vi "AIDI-Initialize DI.vi"(0 "DI":T2, 7 "Sync Task":refnum<k21>, 11 "error in (no error)":errorcluster) -> (4 "DI Tasks":T1, 15 "error out":errorcluster)   [LabVIEW 2020]
uses:
  Typedefs/DI-Output Spec.ctl
  Typedefs/AIDI-DI Tasks.ctl
  <resource>/objmgr/daqmx.rc
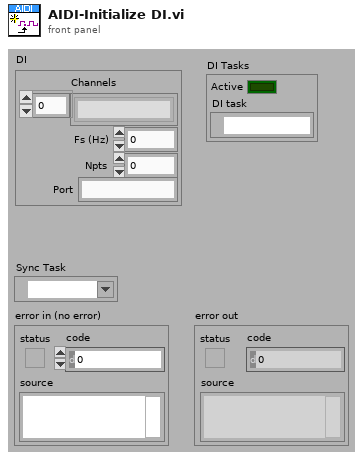
[diagram p1: front panel]
types:
  T1 = typedef "AIDI-DI Tasks.ctl" = cluster{"Active":bool, "DI task":refnum<k21>}
  T2 = typedef "DI-Output Spec.ctl" = cluster{"Channels":string[], "Fs (Hz)":dbl, "Npts":i32, "Port":string}
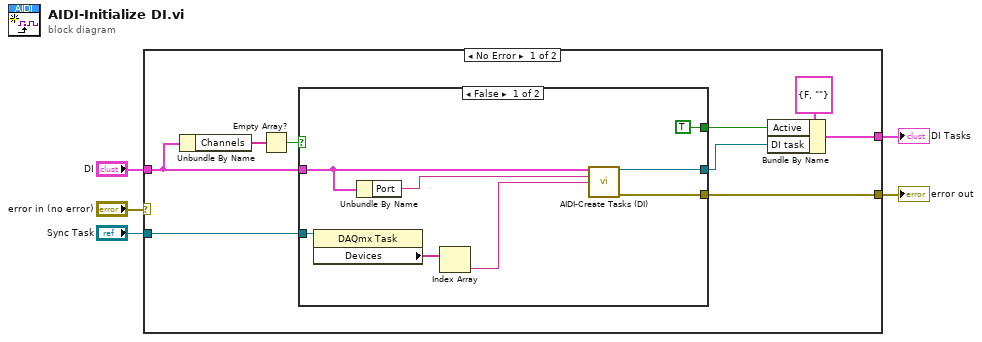
[diagram p0: block diagram]
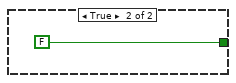
[diagram p2: hidden frame]
diagram:
  n1 = case shown="No Error" "error in (no error)" {
    selector: "error in (no error)" -> [_ w24]
    tunnel: [w14 w24] -> w5
    tunnel: "DI" -> [w12 _]
    tunnel: "Sync Task" -> [w13 _]
    tunnel: [w7 _] -> w1
    frame No Error {
      n2 = Unbundle By Name(w12) -> ("Channels"=w11:string[])
      n3 = Empty Array?(array=w11) -> (empty?=w10:bool)
      n4 = case shown="False" w10 {
        tunnel: [w18 _] -> w14
        tunnel: w13 -> [w17 _]
        tunnel: w12 -> [w21 _]
        tunnel: [w19 _] -> w9
        tunnel: [TRUE FALSE] -> w8
        frame False {
          n5 = property class="DAQmx Task"(reference=w17) -> ("Devices"=w16:tag[])  [unwired: 1 in, 2 out]
          n6 = Unbundle By Name(w21) -> ("Port"=w20:string)
          n7 = Index Array(array=w16) -> (element=w15:tag)  [unwired: 1 in]
          n8 = call "AIDI-Create Tasks (DI).vi"("DI"=w21, "DI Device Name"=w20, "Sync Device Name"=w15) -> ("task out"=w19:refnum<k21>, "error out"=w18:errorcluster)  [unwired: 11 in]
        }
        frame True {
        }
      }
      n9 = Bundle By Name(cluster=T1 {"Active"=FALSE, "DI task"=""} ("DO Tasks"), "Active"=w8, "DI task"=w9) -> (w7:T1)
    }
    frame Error {
    }
  }
  "error out" <- w5
  "DI Tasks" <- w1
